vi "CoordToMeters.vi"(9 "VelNed":cluster{"North":dbl, "East":dbl, "Down":dbl} {"Down" format="%#.11g"; "East" format="%#.11g"; "North" format="%#.11g"}, 10 "Ref Point":cluster{"Lat":dbl, "Long":dbl} {"Long" format="%#.22g"; "Lat" format="%#.22g"}, 11 "GPS position":cluster{"Lat":dbl, "Long":dbl} {"Long" format="%#.22g"; "Lat" format="%#.22g"}) -> (1 "Bike Heading":dbl, 2 "X":dbl format="%#.14g", 3 "Y":dbl format="%#.14g")   [LabVIEW 2016]
uses:
  <vilib>/imath/engines/lvmath2/RunTimeEngine/NodeEndStatement/NIMS_NodeEndStatement_Output.vi
  <instcachedir>/0/NIMS_NodeEndStatement_Output_53EC0D466D134D7ABD903AC30B43404B.lvgen/NIMS_NodeEndStatement_Output_53EC0D466D134D7ABD903AC30B43404B_001.vi
  <vilib>/imath/engines/lvmath2/RunTimeEngine/ErrorHandling/NIMS_Finalize Error.vi
panel:
  out "Distance to the reference point":dbl format="%#.22g"
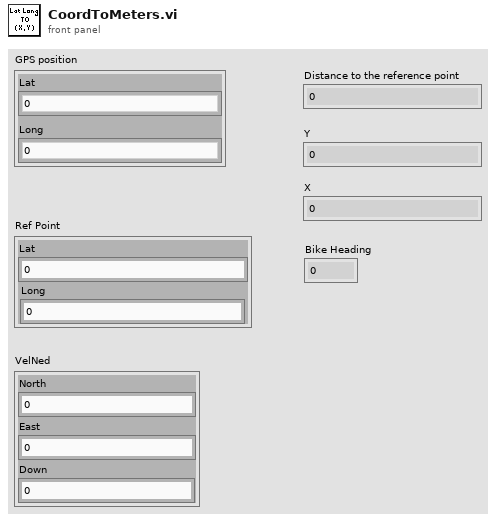
[diagram p1: front panel]
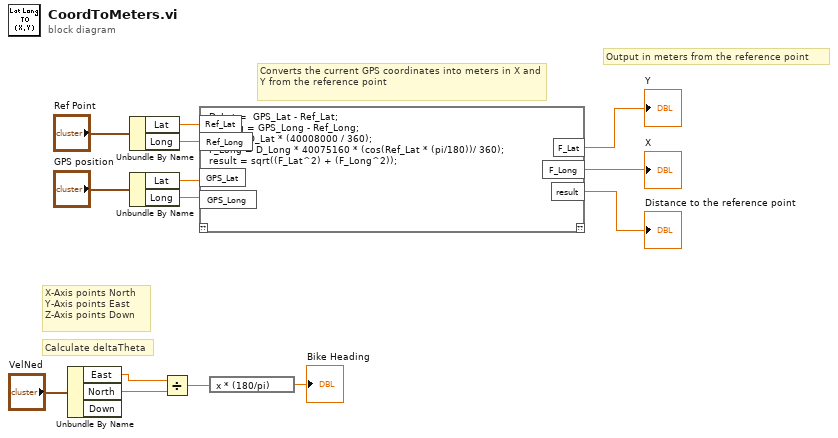
[diagram p0: block diagram]
diagram:
  # "Calculate deltaTheta"
  # "X-Axis points North\nY-Axis points East\nZ-Axis points Down"
  # "Output in meters from the reference point"
  # "Converts the current GPS coordinates into meters in X and Y from the reference point"
  n1 = Unbundle By Name("VelNed") -> ("East"=w4:dbl, "North"=w3:dbl)  [unwired: 1 out]
  n2 = Unbundle By Name("Ref Point") -> ("Lat"=w11:dbl, "Long"=w10:dbl)
  n3 = Unbundle By Name("GPS position") -> ("Lat"=w7:dbl, "Long"=w6:dbl)
  n4 = Divide(x=w4, y=w3) -> (x/y=w2:dbl)
  n5 = mathscript code="D_Lat =  GPS_Lat - Ref_Lat;\nD_Long = GPS_Long - Ref_Long;\nF_Lat = D_Lat * (40008000 / 360);\nF_Long = D_Long * 40075160 * (cos(Ref_Lat * (pi/180))/ 360);\nresult = sqrt((F_Lat^2) + (F_Long^2));"("Ref_Lat"=w11, "Ref_Long"=w10, "GPS_Lat"=w7, "GPS_Long"=w6) -> ("result"=→"Distance to the reference point":dbl, "F_Lat"=→"Y":dbl, "F_Long"=→"X":dbl)  [unwired: 1 in, 1 out]
  n6 = expression code="x * (180/pi)"(w2) -> (→"Bike Heading":dbl)
